vi "Popup Borders.vi"(10 "Row":cluster{"#":i16, "to #":i16}, 11 "VI refnum":refnum<vi>) -> ()   [LabVIEW 2013]
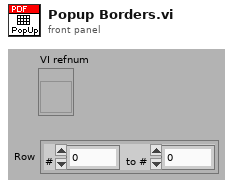
[diagram p1: front panel]
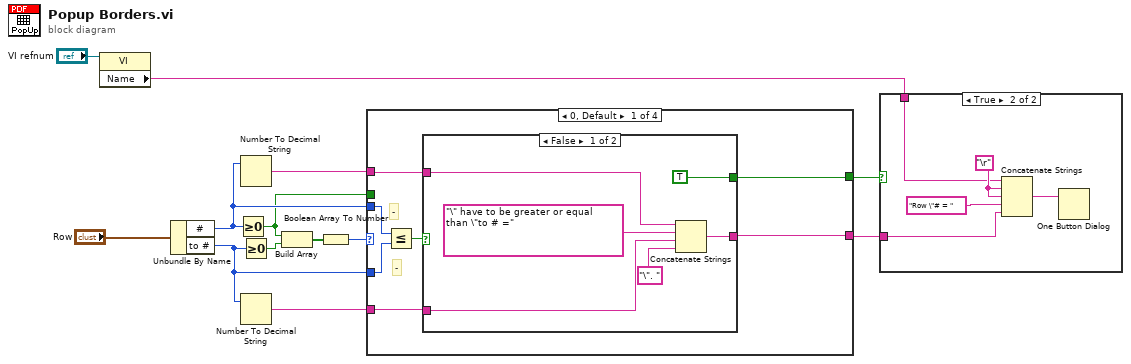
[diagram p0: block diagram]
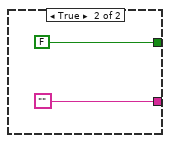
[diagram p2: hidden frame]
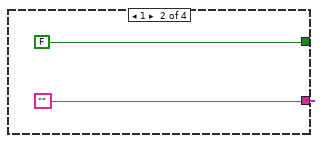
[diagram p3: hidden frame]
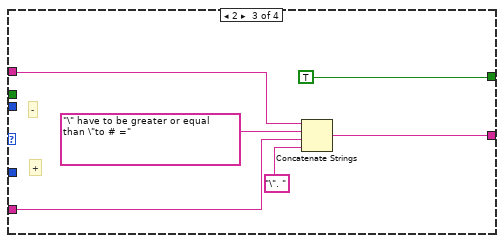
[diagram p4: hidden frame]
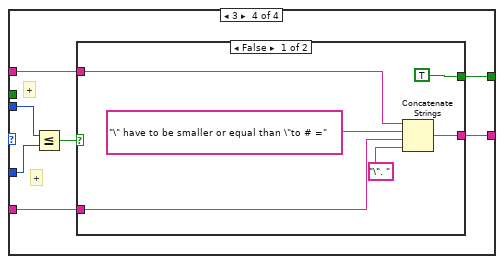
[diagram p5: hidden frame]
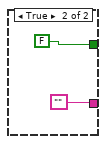
[diagram p6: hidden frame]
diagram:
  n1 = property class="VI"(reference="VI refnum") -> ("Name"=w13:string)  [unwired: 1 in, 2 out]
  n2 = Unbundle By Name("Row") -> ("#"=w8:i16, "to #"=w7:i16)
  n3 = Greater Or Equal To 0?(x=w8) -> (x >= 0?=w4:bool)
  n4 = Number To Decimal String(number=w8) -> (decimal integer string=w6:string)  [unwired: 1 out]
  n5 = Greater Or Equal To 0?(x=w7) -> (x >= 0?=w10:bool)
  n6 = Number To Decimal String(number=w7) -> (decimal integer string=w5:string)  [unwired: 1 out]
  n7 = Build Array(w4, w10) -> (w11:bool[])
  n8 = Boolean Array To Number(Boolean array=w11) -> (number=w9:u32)
  n9 = case shown="0, Default" w9 {
    tunnel: w8 -> [w19 _ _ w42]
    tunnel: w7 -> [w20 _ _ w43]
    tunnel: w6 -> [w18 _ w36 w40]
    tunnel: w5 -> [w17 _ w35 w39]
    tunnel: [w15 FALSE TRUE w38] -> w3
    tunnel: [w14 "" w33 w37] -> w2
    tunnel: w4 -> [_ _ _ _]
    frame 0, Default {
      # "-"
      # "-"
      n10 = Less Or Equal?(x=w19, y=w20) -> (x <= y?=w16:bool)
      n11 = case shown="False" w16 {
        tunnel: [TRUE FALSE] -> w15
        tunnel: [w22 ""] -> w14
        tunnel: w18 -> [w24 _]
        tunnel: w17 -> [w23 _]
        frame False {
          n12 = Concatenate Strings(w24, "\" have to be greater or equal than \"to # =", w23, "\". ") -> (w22:string)
        }
        frame True {
        }
      }
    }
    frame 1 {
    }
    frame 2 {
      # "+"
      # "-"
      n13 = Concatenate Strings(w36, "\" have to be greater or equal than \"to # =", w35, "\". ") -> (w33:string)
    }
    frame 3 {
      # "+"
      # "+"
      n14 = Less Or Equal?(x=w42, y=w43) -> (x <= y?=w41:bool)
      n15 = case shown="False" w41 {
        tunnel: [TRUE FALSE] -> w38
        tunnel: w40 -> [w47 _]
        tunnel: w39 -> [w46 _]
        tunnel: [w45 ""] -> w37
        frame False {
          n16 = Concatenate Strings(w47, "\" have to be smaller or equal than \"to # =", w46, "\". ") -> (w45:string)
        }
        frame True {
        }
      }
    }
  }
  n17 = case shown="True" w3 {
    tunnel: w13 -> [_ w54]
    tunnel: w2 -> [_ w52]
    frame False {
    }
    frame True {
      w55 = "\r"
      n18 = Concatenate Strings(w54, w55, w55, "Row \"# = ", w52) -> (w56:string)
      n19 = One Button Dialog(message=w56) -> ()  [unwired: 2 out]
    }
  }
